vi "number2-calculator.vi"() -> ()   [LabVIEW 2014]
panel:
  in  "Stop Button":bool
  in  "1":bool
  in  "2":bool
  in  "3":bool
  in  "4":bool
  in  "+":bool
  in  "=":bool
  in  "7":bool
  in  "0":bool
  in  "5":bool
  in  "9":bool
  in  "8":bool
  in  "6":bool
  in  "-":bool
  in  "⊙":bool
  in  "∫":bool
  in  ".":bool
  in  "c":bool
  in  "Backspace":bool
  in  "String":string
  in  "String 2":string
  in  "String 3":string
  out "Numeric":i32=1
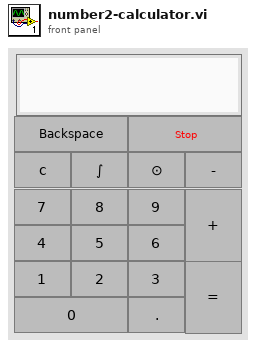
[diagram p1: front panel]
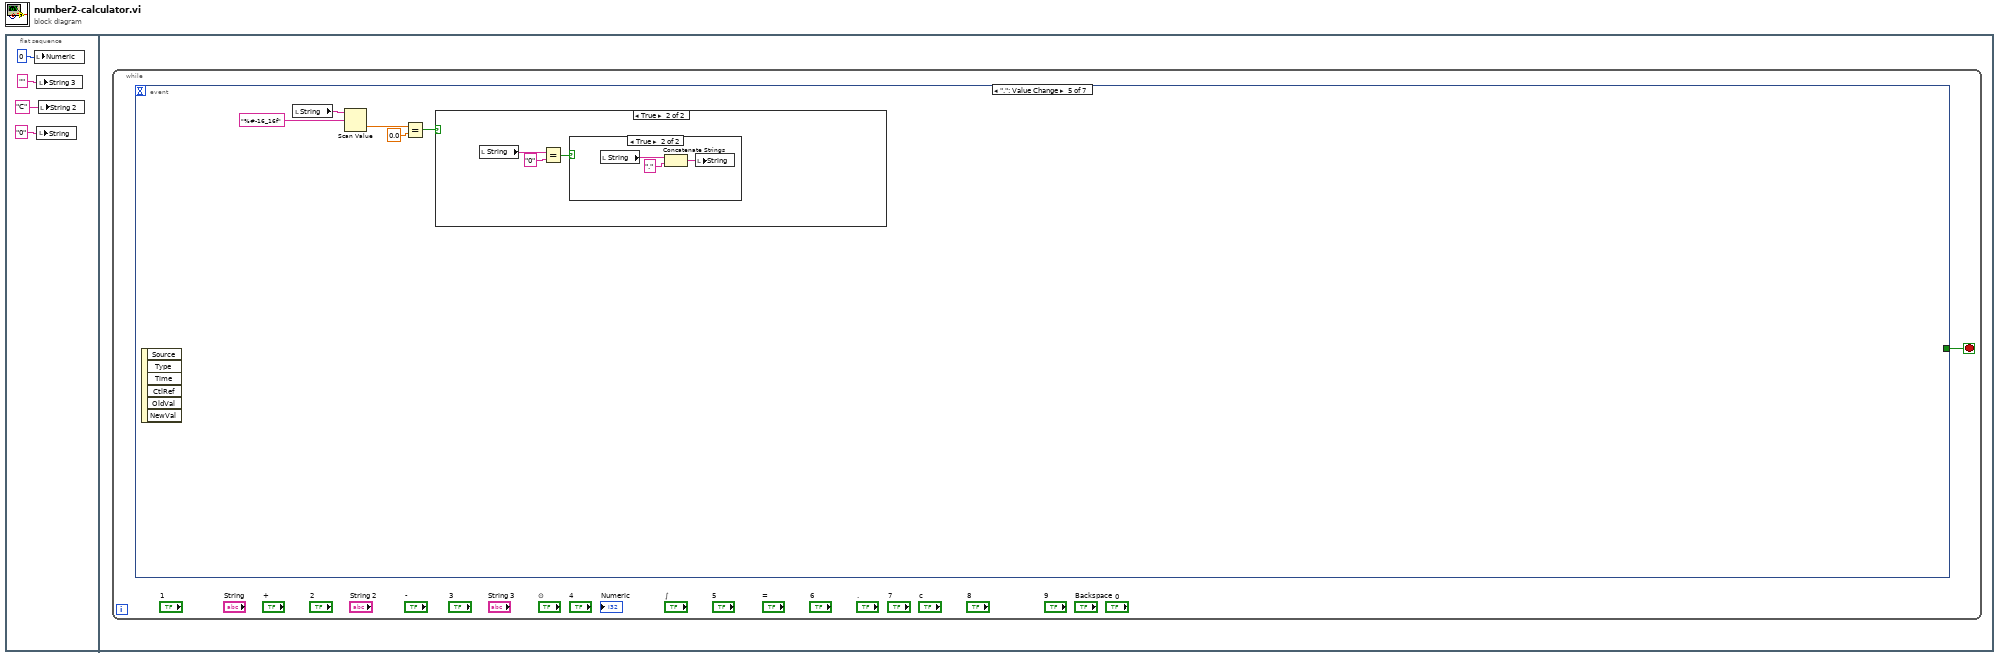
[diagram p0: block diagram]
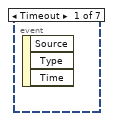
[diagram p2: hidden frame]
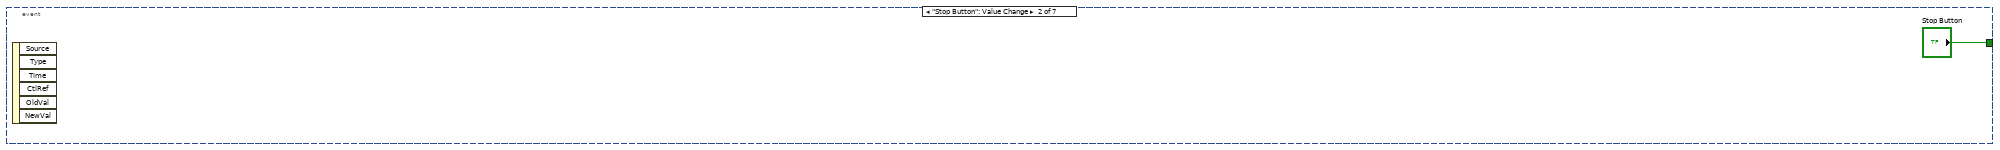
[diagram p3: hidden frame]
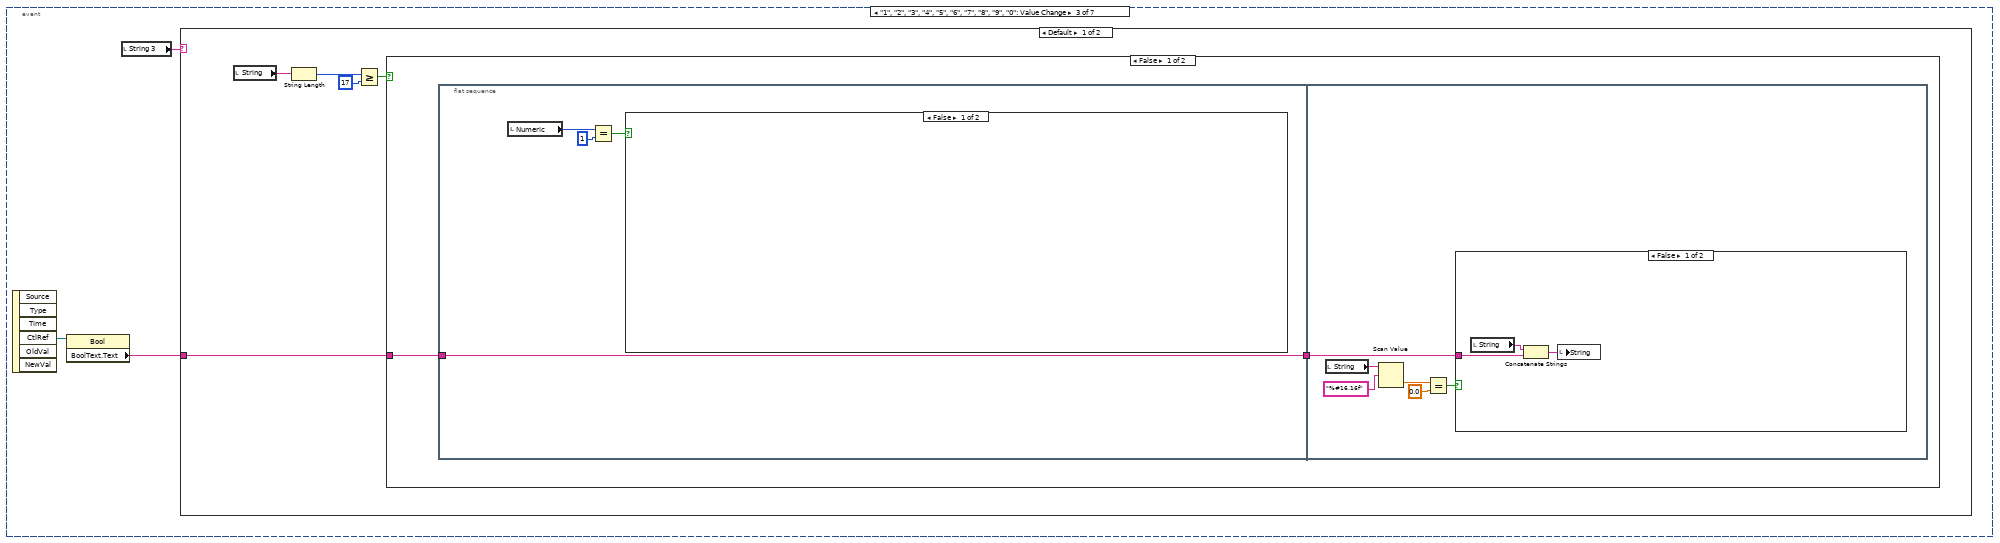
[diagram p4: hidden frame]
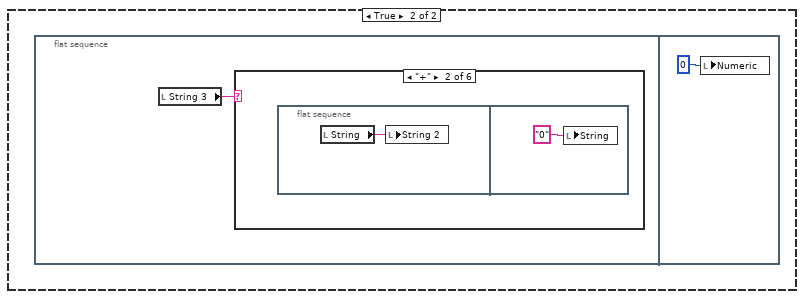
[diagram p5: hidden frame]
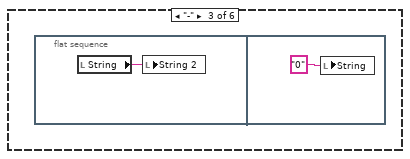
[diagram p7: hidden frame]
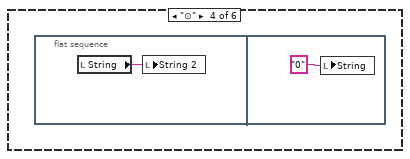
[diagram p8: hidden frame]
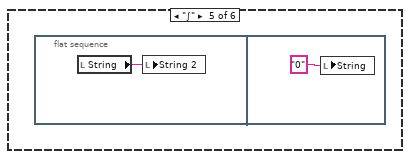
[diagram p9: hidden frame]
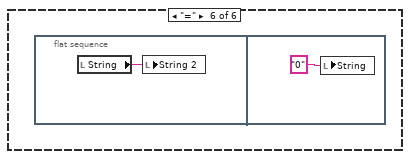
[diagram p10: hidden frame]
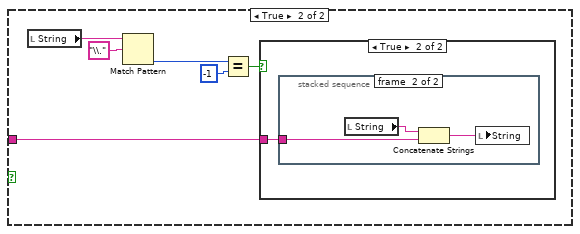
[diagram p11: hidden frame]
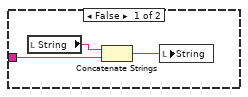
[diagram p12: hidden frame]
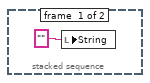
[diagram p13: hidden frame]
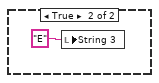
[diagram p14: hidden frame]
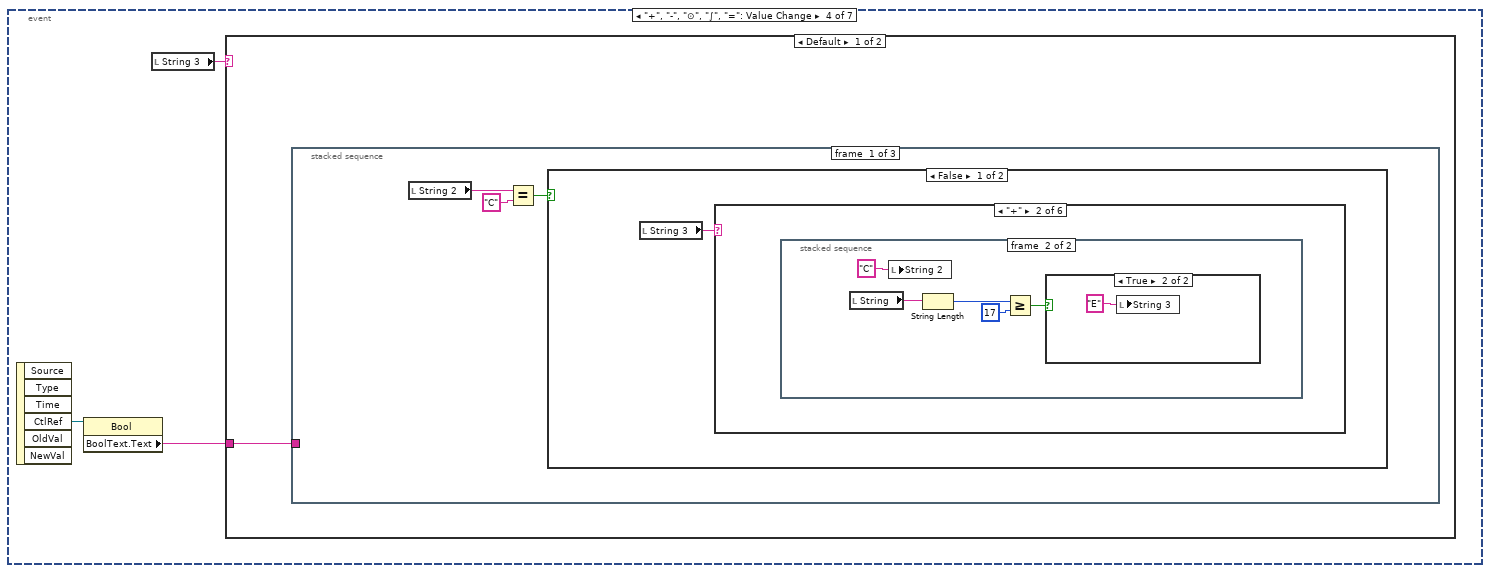
[diagram p16: hidden frame]
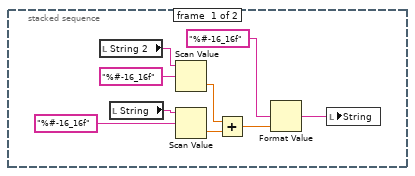
[diagram p18: hidden frame]
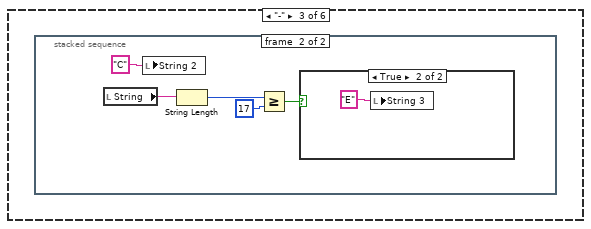
[diagram p20: hidden frame]
diagram:
  n1 = flat-sequence {
    frame #0 {
      n2 = local write "Numeric"(0 ("Numeric")) -> ()
      n3 = local write "String 3"("") -> ()
      n4 = local write "String"("0") -> ()
      n5 = local write "String 2"("C") -> ()
    }
    frame #1 {
      n6 = while {
        stop <- w5 stop-if-true
        n7 = event shown="[4] \".\": Value Change" {
          selector: _ -> [_ _ _ _ _ _ _]
          dyn-events: _ -> [_ _ _ _ _ _ _]
          timeout: _ -> [_ _ _ _ _ _ _]
          tunnel: [_ "Stop Button" _ _ _ _ _] -> w5
          event Timeout {
            n8 = event-data() -> ()  [unwired: 1 in, 3 out]
          }
          event "Stop Button": Value Change {
            n9 = event-data() -> ()  [unwired: 1 in, 6 out]
          }
          event "1", "2", "3", "4", "5", "6", "7", "8", "9", "0": Value Change {
            n10 = event-data() -> ("CtlRef"=w9:refnum<vi>)  [unwired: 1 in, 5 out]
            n11 = property class="Bool"(reference=w9) -> ("BoolText.Text"=w7:string)  [unwired: 1 in, 2 out]
            n12 = local read "String 3"() -> (w8:string)
            n13 = case shown="Default" w8 {
              tunnel: w7 -> [w10 _]
              frame Default {
                n14 = local read "String"() -> (w14:string)
                n15 = String Length(string=w14) -> (length=w13:i32)
                n16 = Greater Or Equal?(x=w13, y=17) -> (x >= y?=w11:bool)
                n17 = case shown="False" w11 {
                  tunnel: w10 -> [w16 _]
                  frame False {
                    n18 = flat-sequence {
                      tunnel: w16 -> [w17]
                      tunnel: [w17] -> w15
                      tunnel: w15 -> [w36]
                      frame #0 {
                        n19 = local read "Numeric"() -> (w19:i32)
                        n20 = Equal?(x=w19, y=1) -> (x = y?=w20:bool)
                        n21 = case shown="False" w20 {
                          frame False {
                          }
                          frame True {
                            n22 = flat-sequence {
                              frame #0 {
                                n23 = local read "String 3"() -> (w21:string)
                                n24 = case shown="\"+\"" w21 {
                                frame Default {
                                }
                                frame "+" {
                                n25 = flat-sequence {
                                frame #0 {
                                n26 = local read "String"() -> (w22:string)
                                n27 = local write "String 2"(w22) -> ()
                                }
                                frame #1 {
                                n28 = local write "String"("0") -> ()
                                }
                                }
                                }
                                frame "-" {
                                n29 = flat-sequence {
                                frame #0 {
                                n30 = local read "String"() -> (w24:string)
                                n31 = local write "String 2"(w24) -> ()
                                }
                                frame #1 {
                                n32 = local write "String"("0") -> ()
                                }
                                }
                                }
                                frame "⊙" {
                                n33 = flat-sequence {
                                frame #0 {
                                n34 = local read "String"() -> (w26:string)
                                n35 = local write "String 2"(w26) -> ()
                                }
                                frame #1 {
                                n36 = local write "String"("0") -> ()
                                }
                                }
                                }
                                frame "∫" {
                                n37 = flat-sequence {
                                frame #0 {
                                n38 = local read "String"() -> (w28:string)
                                n39 = local write "String 2"(w28) -> ()
                                }
                                frame #1 {
                                n40 = local write "String"("0") -> ()
                                }
                                }
                                }
                                frame "=" {
                                n41 = flat-sequence {
                                frame #0 {
                                n42 = local read "String"() -> (w30:string)
                                n43 = local write "String 2"(w30) -> ()
                                }
                                frame #1 {
                                n44 = local write "String"("0") -> ()
                                }
                                }
                                }
                                }
                              }
                              frame #1 {
                                n45 = local write "Numeric"(0) -> ()
                              }
                            }
                          }
                        }
                      }
                      frame #1 {
                        n46 = local read "String"() -> (w35:string)
                        n47 = Scan Value(string=w35, format string="%#16.16f") -> (value=w33:dbl)  [unwired: 1 in, 1 out]
                        n48 = Equal?(x=w33, y=0.0) -> (x = y?=w38:bool)
                        n49 = case shown="False" w38 {
                          tunnel: w36 -> [w39 w42]
                          frame False {
                            n50 = local read "String"() -> (w41:string)
                            n51 = Concatenate Strings(w41, w39) -> (w40:string)
                            n52 = local write "String"(w40) -> ()
                          }
                          frame True {
                            n53 = local read "String"() -> (w44:string)
                            n54 = Match Pattern(string=w44, regular expression="\\.") -> (offset past match=w46:i32)  [unwired: 1 in, 3 out]
                            n55 = Equal?(x=w46, y=-1) -> (x = y?=w43:bool)
                            n56 = case shown="True" w43 {
                              tunnel: w42 -> [w48 w51]
                              frame False {
                                n57 = local read "String"() -> (w49:string)
                                n58 = Concatenate Strings(w49, w48) -> (w50:string)
                                n59 = local write "String"(w50) -> ()
                              }
                              frame True {
                                n60 = stacked-sequence {
                                tunnel: w51 -> [_ w53]
                                frame #0 {
                                n61 = local write "String"("") -> ()
                                }
                                frame #1 {
                                n62 = local read "String"() -> (w55:string)
                                n63 = Concatenate Strings(w55, w53) -> (w54:string)
                                n64 = local write "String"(w54) -> ()
                                }
                                }
                              }
                            }
                          }
                        }
                      }
                    }
                  }
                  frame True {
                    n65 = local write "String 3"("E") -> ()
                  }
                }
              }
              frame "E" {
              }
            }
          }
          event "+", "-", "⊙", "∫", "=": Value Change {
            n66 = event-data() -> ("CtlRef"=w59:refnum<vi>)  [unwired: 1 in, 5 out]
            n67 = property class="Bool"(reference=w59) -> ("BoolText.Text"=w57:string)  [unwired: 1 in, 2 out]
            n68 = local read "String 3"() -> (w58:string)
            n69 = case shown="Default" w58 {
              tunnel: w57 -> [w60 _]
              frame Default {
                n70 = stacked-sequence {
                  tunnel: w60 -> [_ _ w132]
                  frame #0 {
                    n71 = local read "String 2"() -> (w61:string)
                    n72 = Equal?(x=w61, y="C") -> (x = y?=w63:bool)
                    n73 = case shown="False" w63 {
                      frame False {
                        n74 = local read "String 3"() -> (w64:string)
                        n75 = case shown="\"+\"" w64 {
                          frame Default {
                          }
                          frame "+" {
                            n76 = stacked-sequence {
                              frame #0 {
                                n77 = local read "String 2"() -> (w73:string)
                                n78 = local read "String"() -> (w72:string)
                                n79 = Scan Value(string=w73, format string="%#-16_16f") -> (value=w71:dbl)  [unwired: 1 in, 1 out]
                                n80 = Scan Value(string=w72, format string="%#-16_16f") -> (value=w70:dbl)  [unwired: 1 in, 1 out]
                                n81 = Add(x=w71, y=w70) -> (x+y=w69:dbl)
                                n82 = Format Value(format string="%#-16_16f", value (0)=w69) -> (output string=w68:string)  [unwired: 1 in]
                                n83 = local write "String"(w68) -> ()
                              }
                              frame #1 {
                                n84 = local read "String"() -> (w77:string)
                                n85 = local write "String 2"("C") -> ()
                                n86 = String Length(string=w77) -> (length=w76:i32)
                                n87 = Greater Or Equal?(x=w76, y=17) -> (x >= y?=w74:bool)
                                n88 = case shown="True" w74 {
                                frame False {
                                }
                                frame True {
                                n89 = local write "String 3"("E") -> ()
                                }
                                }
                              }
                            }
                          }
                          frame "-" {
                            n90 = stacked-sequence {
                              frame #0 {
                                n91 = local read "String 2"() -> (w88:string)
                                n92 = local read "String"() -> (w87:string)
                                n93 = Scan Value(string=w88, format string="%#-16_16f") -> (value=w86:dbl)  [unwired: 1 in, 1 out]
                                n94 = Scan Value(string=w87, format string="%#-16_16f") -> (value=w85:dbl)  [unwired: 1 in, 1 out]
                                n95 = Subtract(x=w86, y=w85) -> (x-y=w84:dbl)
                                n96 = Format Value(format string="%#-16_16f", value (0)=w84) -> (output string=w83:string)  [unwired: 1 in]
                                n97 = local write "String"(w83) -> ()
                              }
                              frame #1 {
                                n98 = local read "String"() -> (w92:string)
                                n99 = local write "String 2"("C") -> ()
                                n100 = String Length(string=w92) -> (length=w91:i32)
                                n101 = Greater Or Equal?(x=w91, y=17) -> (x >= y?=w89:bool)
                                n102 = case shown="True" w89 {
                                frame False {
                                }
                                frame True {
                                n103 = local write "String 3"("E") -> ()
                                }
                                }
                              }
                            }
                          }
                          frame "⊙" {
                            n104 = stacked-sequence {
                              frame #0 {
                                n105 = local read "String 2"() -> (w103:string)
                                n106 = local read "String"() -> (w102:string)
                                n107 = Scan Value(string=w103, format string="%#-16_16f") -> (value=w101:dbl)  [unwired: 1 in, 1 out]
                                n108 = Scan Value(string=w102, format string="%#-16_16f") -> (value=w100:dbl)  [unwired: 1 in, 1 out]
                                n109 = Multiply(x=w101, y=w100) -> (x*y=w99:dbl)
                                n110 = Format Value(format string="%#-16_16f", value (0)=w99) -> (output string=w98:string)  [unwired: 1 in]
                                n111 = local write "String"(w98) -> ()
                              }
                              frame #1 {
                                n112 = local read "String"() -> (w107:string)
                                n113 = local write "String 2"("C") -> ()
                                n114 = String Length(string=w107) -> (length=w106:i32)
                                n115 = Greater Or Equal?(x=w106, y=17) -> (x >= y?=w104:bool)
                                n116 = case shown="True" w104 {
                                frame False {
                                }
                                frame True {
                                n117 = local write "String 3"("E") -> ()
                                }
                                }
                              }
                            }
                          }
                          frame "∫" {
                            n118 = stacked-sequence {
                              frame #0 {
                                n119 = local read "String 2"() -> (w118:string)
                                n120 = local read "String"() -> (w116:string)
                                n121 = Scan Value(string=w118, format string="%#-16_16f") -> (value=w114:dbl)  [unwired: 1 in, 1 out]
                                n122 = Scan Value(string=w116, format string="%#-16_16f") -> (value=w113:dbl)  [unwired: 1 in, 1 out]
                                n123 = Divide(x=w114, y=w113) -> (x/y=w112:dbl)
                                n124 = Format Value(format string="%#-16_16f", value (0)=w112) -> (output string=w111:string)  [unwired: 1 in]
                                n125 = local write "String"(w111) -> ()
                              }
                              frame #1 {
                                n126 = local read "String"() -> (w122:string)
                                n127 = local write "String 2"("C") -> ()
                                n128 = String Length(string=w122) -> (length=w121:i32)
                                n129 = Greater Or Equal?(x=w121, y=17) -> (x >= y?=w119:bool)
                                n130 = case shown="True" w119 {
                                frame False {
                                }
                                frame True {
                                n131 = local write "String 3"("E") -> ()
                                }
                                }
                              }
                            }
                          }
                          frame "=" {
                          }
                        }
                      }
                      frame True {
                      }
                    }
                  }
                  frame #1 {
                    n132 = local read "String 3"() -> (w125:string)
                    n133 = case shown="\"⊙\"" w125 {
                      frame Default {
                      }
                      frame "+" {
                        n134 = local write "String 3"("") -> ()
                      }
                      frame "-" {
                        n135 = local write "String 3"("") -> ()
                      }
                      frame "⊙" {
                        n136 = local write "String 3"("") -> ()
                      }
                      frame "∫" {
                        n137 = local write "String 3"("") -> ()
                      }
                      frame "=" {
                        n138 = local write "String 3"("") -> ()
                      }
                      frame "E" {
                      }
                    }
                  }
                  frame #2 {
                    n139 = local read "String 3"() -> (w131:string)
                    n140 = case shown="Default" w131 {
                      tunnel: w132 -> [w133 _]
                      frame Default {
                        n141 = local read "String 3"() -> (w135:string)
                        n142 = local write "Numeric"(1) -> ()
                        n143 = Concatenate Strings(w135, w133) -> (w136:string)
                        n144 = local write "String 3"(w136) -> ()
                      }
                      frame "E" {
                      }
                    }
                  }
                }
              }
              frame "E" {
              }
            }
          }
          event ".": Value Change {
            n145 = event-data() -> ()  [unwired: 1 in, 6 out]
            n146 = local read "String"() -> (w139:string)
            n147 = Scan Value(string=w139, format string="%#-16_16f") -> (value=w137:dbl)  [unwired: 1 in, 1 out]
            n148 = Equal?(x=w137, y=0.0) -> (x = y?=w141:bool)
            n149 = case shown="True" w141 {
              frame False {
                n150 = local read "String"() -> (w142:string)
                n151 = Match Pattern(string=w142, regular expression="\\.") -> (offset past match=w145:i32)  [unwired: 1 in, 3 out]
                n152 = Equal?(x=w145, y=-1) -> (x = y?=w143:bool)
                n153 = case shown="True" w143 {
                  frame False {
                  }
                  frame True {
                    n154 = local read "String"() -> (w149:string)
                    n155 = Concatenate Strings(w149, ".") -> (w147:string)
                    n156 = local write "String"(w147) -> ()
                  }
                }
              }
              frame True {
                n157 = local read "String"() -> (w151:string)
                n158 = Equal?(x=w151, y="0") -> (x = y?=w152:bool)
                n159 = case shown="True" w152 {
                  frame False {
                  }
                  frame True {
                    n160 = local read "String"() -> (w153:string)
                    n161 = Concatenate Strings(w153, ".") -> (w155:string)
                    n162 = local write "String"(w155) -> ()
                  }
                }
              }
            }
          }
          event "Backspace": Value Change {
            n163 = event-data() -> ()  [unwired: 1 in, 6 out]
            n164 = local read "String"() -> (w159:string)
            n165 = String Length(string=w159) -> (length=w158:i32)
            n166 = Less Or Equal?(x=w158, y=1) -> (x <= y?=w156:bool)
            n167 = case shown="False" w156 {
              frame False {
                n168 = local read "String"() -> (w163:string)
                n169 = String Length(string=w163) -> (length=w164:i32)
                n170 = Subtract(x=w164, y=1) -> (x-y=w162:i32)
                n171 = String Subset(string=w163, offset (0)=0, length (rest)=w162) -> (substring=w161:string)
                n172 = local write "String"(w161) -> ()
              }
              frame True {
                n173 = local write "String"("0") -> ()
              }
            }
          }
          event "c": Value Change {
            n174 = event-data() -> ()  [unwired: 1 in, 6 out]
            n175 = local write "String"("0") -> ()
            n176 = local read "String 3"() -> (w167:string)
            n177 = case shown="\"=\"" w167 {
              frame Default {
              }
              frame "=" {
                n178 = local write "String 3"("") -> ()
              }
            }
          }
        }
      }
    }
  }
